vi "Module ID.vi"(11 "Data Logger Module in":refnum<class "Data Logger Module.lvclass">) -> (2 "Module ID":string)   [LabVIEW 2020, in "VolatusData.lvlib" / "Data Logger Module.lvclass"]
uses:
  Data Logger Module.lvclass
  Data Logger Module.lvclass/Data Logger Module.ctl
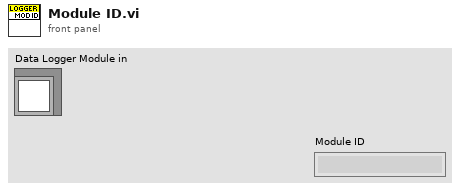
[diagram p1: front panel]
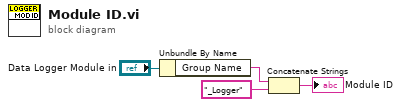
[diagram p0: block diagram]
diagram:
  n1 = Unbundle By Name("Data Logger Module in") -> ("Group Name"=w3:string)
  n2 = Concatenate Strings(w3, "_Logger" ("string")) -> (→"Module ID":string)
